vi "TCP IP Connection Timing Tester.vi"() -> ()   [LabVIEW 2024]
panel:
  out "Array":T1(array[cluster])
  out "output cluster":T2
  out "Fornax Connection out":refnum<k5>
  out "error out":errorcluster
  in  "error in (no error)":errorcluster
  in  "Fornax Executable Path":path=path "C:/Program Files (x86)/Medtronic/Fornax/x86/Fornax.exe"
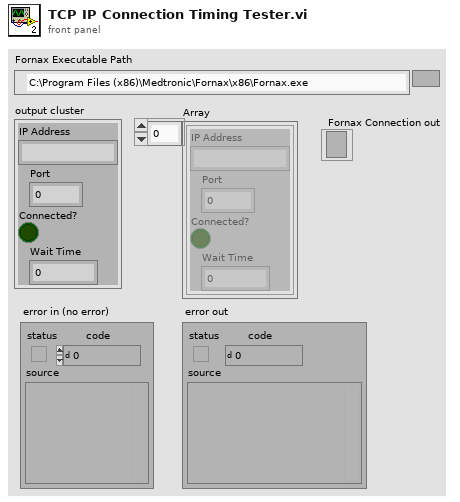
[diagram p1: front panel]
types:
  T1 = cluster{"IP Address":string, "Port":u16, "Connected?":bool, "Wait Time":dbl}[]
  T2 = cluster{"IP Address":string, "Port":u16, "Connected?":bool, "Wait Time":dbl}
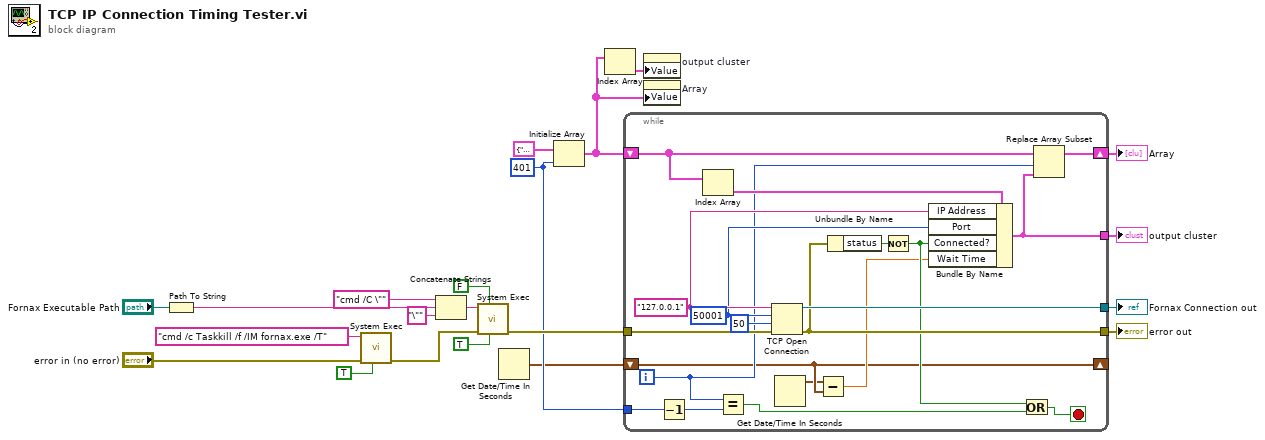
[diagram p0: block diagram]
diagram:
  w16 = 401 ("dimension size")
  n1 = Path To String(path="Fornax Executable Path") -> (string=w5:string)
  n2 = call <vilib>:"System Exec.vi"("run minimized? (F)"=TRUE, "error in (no error)"="error in (no error)", "command line"="cmd /c Taskkill /f /IM fornax.exe /T") -> ("error out"=w11:errorcluster)  [unwired: 5 in, 3 out]
  n3 = Concatenate Strings("cmd /C \"" ("string"), w5, "\"" ("string")) -> (w7:string)
  n4 = call <vilib>:"System Exec.vi"("run minimized? (F)"=TRUE, "wait until completion? (T)"=FALSE, "error in (no error)"=w11, "command line"=w7) -> ("error out"=w21:errorcluster)  [unwired: 4 in, 3 out]
  n5 = Get Date/Time In Seconds() -> (seconds since 1Jan1904=w13:timestamp)
  n6 = Initialize Array(T2 {"IP Address"="", "Port"=0, "Connected?"=FALSE, "Wait Time"=0.0} ("Cluster"), w16) -> (w1:T1)
  n7 = Index Array(array=w1) -> (element=w2:T2)  [unwired: 1 in]
  n8 = while {
    tunnel: [w40] -> w19
    shift-right: [w39] -> w14
    shift-left: w1 -> [w38]
    tunnel: w16 -> [w29]
    tunnel: [w26] -> w15
    shift-right: [w23] -> _
    shift-left: w13 -> [w23]
    tunnel: w21 -> [w41]
    tunnel: [w34] -> w20
    i -> [w25]
    stop <- w31 stop-if-true
    w35 = u16 50001 ("remote port or service name")
    w36 = "127.0.0.1" ("address")
    n9 = Decrement(x=w29) -> (x-1=w28:i32)
    n10 = Index Array(array=w38) -> (element=w37:T2)  [unwired: 1 in]
    n11 = Equal?(x=w25, y=w28) -> (x = y?=w27:bool)
    n12 = TCP Open Connection(address=w36, remote port or service name=w35, timeout ms (60000)=50, error in (no error)=w41) -> (connection ID=w40:refnum<k5>, error out=w34:errorcluster)  [unwired: 1 in]
    n13 = Get Date/Time In Seconds() -> (seconds since 1Jan1904=w22:timestamp)
    n14 = Subtract(x=w22, y=w23) -> (x-y=w24:dbl)
    n15 = Unbundle By Name(w34) -> ("status"=w33:bool)
    n16 = Not(x=w33) -> (.not. x?=w30:bool)
    n17 = Bundle By Name(cluster=w37, "IP Address"=w36, "Port"=w35, "Connected?"=w30, "Wait Time"=w24) -> (w26:T2)
    n18 = Or(x=w30, y=w27) -> (x .or. y?=w31:bool)
    n19 = Replace Array Subset(array=w38, new element=w26, index=w25) -> (w39:T1)
  }
  "error out" <- w20
  "Fornax Connection out" <- w19
  "output cluster" <- w15
  "Array" <- w14
  n20 = property on="output cluster" class="Clust (strict)"("Value"=w2) -> ()  [unwired: 2 in, 2 out]
  n21 = property on="Array" class="Arr (strict)"("Value"=w1) -> ()  [unwired: 2 in, 2 out]
